vi "Bundle Script_Set Method Node.vi"(8 "error in":errorcluster, 10 "Property Array":T1(array[cluster]), 11 "Invoke in":refnum<vi>) -> (0 "error out":errorcluster)   [LabVIEW 2023]
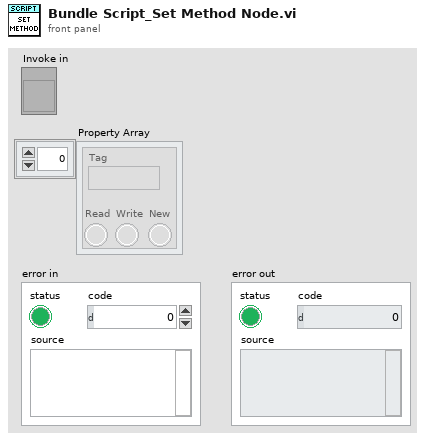
[diagram p1: front panel]
types:
  T1 = cluster{"Tag":string, "Read":bool, "Write":bool, "New":bool}[]
  T2 = cluster{"Tag":string, "Read":bool, "Write":bool, "New":bool}
  T3 = cluster{"Index":u16, "Property Type":enum16{"Unknown", "Base", "Scripting", "Private", "Deprecated", "None", "Divider"}, "ID String":string, "Dotted ID String":string, "Class":string, "Parent":string, "Display name full":string, "Display name short":string, "Parents Array":string[], "Indent":u16}
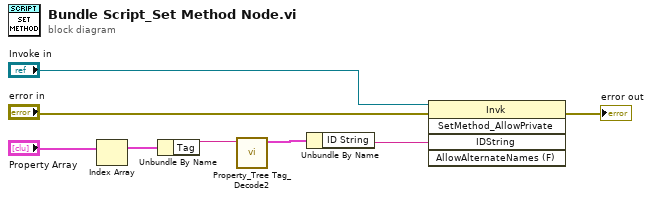
[diagram p0: block diagram]
diagram:
  n1 = Index Array(array="Property Array") -> (element=w7:T2)  [unwired: 1 in]
  n2 = Unbundle By Name(w7) -> ("Tag"=w2:string)
  n3 = call "Property_Tree Tag_Decode2.vi"("Tag In"=w2) -> ("TagData"=w3:T3)  [unwired: 10 in]
  n4 = Unbundle By Name(w3) -> ("ID String"=w1:string)
  n5 = invoke class="Invk" method="SetMethod_AllowPrivate"(reference="Invoke in", error in="error in", "IDString"=w1) -> (error out=→"error out":errorcluster)  [unwired: 2 in, 4 out]
